vi "sedSpectrometer_getSample_spectTemperature.vi"(8 "error in (no error)":errorcluster, 11 "spectTemperature_Ctl":T1) -> (0 "error out":errorcluster, 2 "function return":i32, 3 "spectTemperature_Ctl out":T1)   [LabVIEW 2016, in "SALLV_sedSpectrometer.lvlib"]
doc: "int sedSpectrometer_shm_getSample_spectTemperatureLV(sedSpectrometer_spectTemperatureLV *spectTemperature_Ctl );"
uses:
  SALLV_sedSpectrometer.lvlib
  DataTypes/spectTemperature.ctl
  SALLV_sedSpectrometer.so
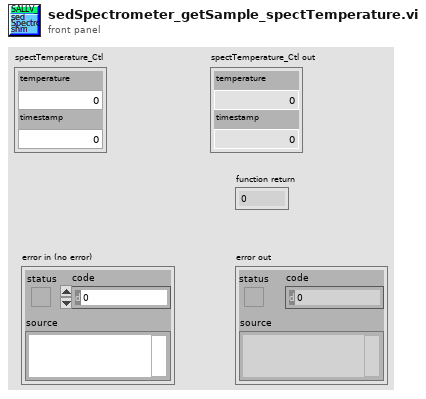
[diagram p1: front panel]
types:
  T1 = typedef "SALLV_sedSpectrometer.lvlib/spectTemperature.ctl" = cluster{"temperature":dbl, "timestamp":dbl}
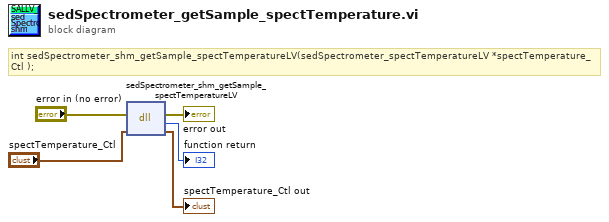
[diagram p0: block diagram]
diagram:
  # "int sedSpectrometer_shm_getSample_spectTemperatureLV(sedSpectrometer_spectTemperatureLV *spectTemperature_Ctl );"
  n1 = dll-call lib="home/harini/TCS/ts_sallv_sedSpectrometer_371/SALLV_sedSpectrometer.*" fn="sedSpectrometer_shm_getSample_spectTemperatureLV"(error in="error in (no error)", "spectTemperature_Ctl"="spectTemperature_Ctl") -> (error out=→"error out":errorcluster, →"function return":i32, "spectTemperature_Ctl"=→"spectTemperature_Ctl out":T1)  [unwired: 2 in, 1 out]
